vi "display-message.vi"(7 "Message Type (0=Progress bar)":i32, 8 "error in (no error)":errorcluster, 9 "Time to wait (x*100ms)":i32=10, 10 "Message":string, 11 "Window Msg in":refnum<class "Window Msg.lvclass">) -> (0 "error out":errorcluster, 3 "Window Msg out":refnum<class "Window Msg.lvclass">)   [LabVIEW 2020]
uses:
  _Common_Lib/UI/Window Msg/Window Msg.lvclass
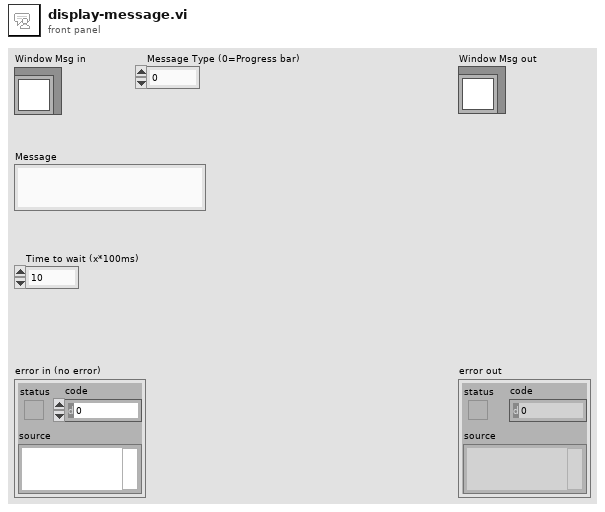
[diagram p1: front panel]
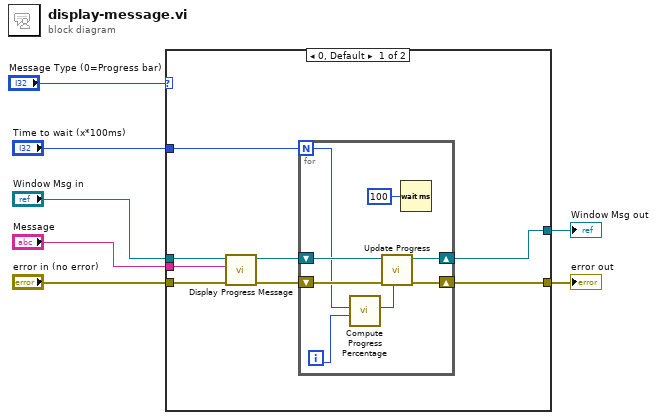
[diagram p0: block diagram]
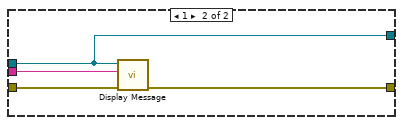
[diagram p2: hidden frame]
diagram:
  n1 = case shown="0, Default" "Message Type (0=Progress bar)" {
    tunnel: "Time to wait (x*100ms)" -> [w13 _]
    tunnel: "Window Msg in" -> [w12 w25]
    tunnel: [w11 w25] -> w5
    tunnel: "Message" -> [w10 w24]
    tunnel: "error in (no error)" -> [w9 w27]
    tunnel: [w8 w26] -> w2
    frame 0, Default {
      n2 = call "Display Progress Message.vi"("error in (no error)"=w9, "Message"=w10, "Window Msg in"=w12) -> ("error out"=w14:errorcluster, "Window Msg out"=w15:refnum<class "Window Msg.lvclass">)  [unwired: 7 in]
      n3 = for {
        N: w13 -> [w18]
        shift-right: [w22] -> w8
        shift-left: w14 -> [w23]
        shift-right: [w20] -> w11
        shift-left: w15 -> [w21]
        i -> [w17]
        n4 = call "Compute Progress Percentage.vi"("Current Iteration"=w17, "Total no. of Iterations"=w18) -> ("Progress Value (%)"=w16:u8)  [unwired: 9 in]
        n5 = call "Update Progress.vi"("Progress"=w16, "error in (no error)"=w23, "Window Msg in"=w21) -> ("error out"=w22:errorcluster, "Window Msg out"=w20:refnum<class "Window Msg.lvclass">)  [unwired: 7 in]
        n6 = Wait (ms)(milliseconds to wait=u32 100) -> ()  [unwired: 1 out]
      }
    }
    frame 1 {
      n7 = call "Display Message.vi"("error in (no error)"=w27, "Message"=w24, "Window Msg in"=w25) -> ("error out"=w26:errorcluster)  [unwired: 8 in]
    }
  }
  "error out" <- w2
  "Window Msg out" <- w5
